vi "AssembleBLMultiplotScript-UandTI.vi"(0 "name or relative path":string, 1 "Final Title":string, 2 "Spectra?":bool, 3 "NormaliseHeight?":bool, 4 "Zref":dbl, 5 "Fit Zmax":dbl, 6 "Fit Zmin":dbl, 7 "HeightJitter%":dbl, 8 "Scale":dbl, 9 "BL Targets":T2[](array[typedef]) {"n" min=0.02 max=0.5 step=0.01 format="%.2f"}, 10 "U,L(U)":refnum<vi>, 11 "UtargetsInfo":T1(array[cluster]), 12 "TI,Sigma":refnum<vi>, 13 "TItargetsInfo":T1(array[cluster]), 15 "No d0":cluster{"n":dbl, "d0":dbl, "d0 2":dbl}, 17 "with d0":cluster{"n":dbl, "d0":dbl, "d0 2":dbl}) -> (20 "gnuplotOut":string)   [LabVIEW 2014]
uses:
  EnFloSFCPPHybrid/Anemometry/Anemometry Sub Vis/Data_plotting_vis/gnuplotScriptComponents/BLPlottersubVIs/BLTarget.ctl
  EnFloSFCPPHybrid/Anemometry/Anemometry Sub Vis/Data_plotting_vis/gnuplotScriptComponents/at.ctl
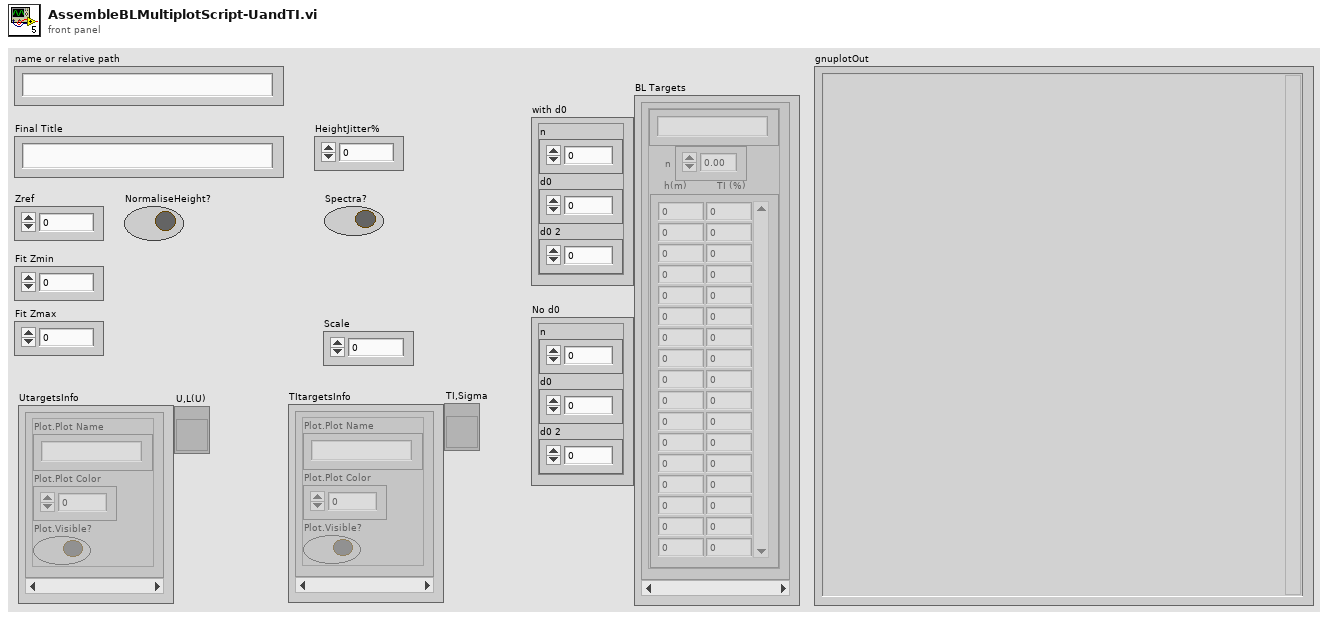
[diagram p1: front panel]
types:
  T1 = cluster{"Plot.Plot Name":string, "Plot.Plot Color":u32, "Plot.Visible?":bool}[]
  T2 = typedef "BLTarget.ctl" = cluster{"Code":string, "TI Profile (FS)":dbl[][], "n":dbl}
  T3 = typedef "at.ctl" = cluster{"XcoordSys":string, "YcoordSys":string, "Xvalue":dbl, "Yvalue":dbl}
  T4 = typedef "minAndMax.ctl" = cluster{"Min":T5, "Max":T5}
  T5 = typedef "AutoManualNumber.ctl" = cluster{"Auto":bool, "Value":dbl}
  T6 = cluster{"No d0":cluster{"n":dbl, "d0":dbl, "d0 2":dbl}, "with d0":cluster{"n":dbl, "d0":dbl, "d0 2":dbl}}
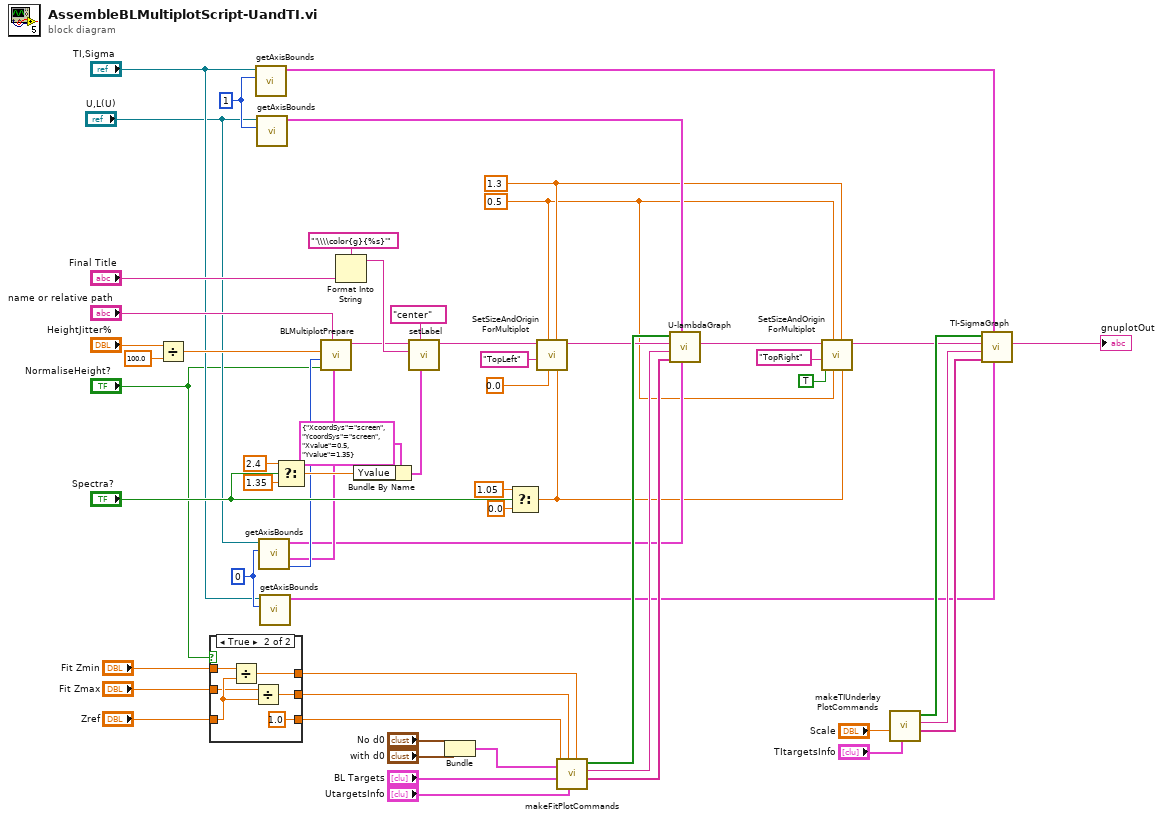
[diagram p0: block diagram]
diagram:
  w16 = 0.5 ("IndividualWidth")
  w17 = 1.3 ("IndividualHeight")
  w11 = 1 ("Active X Scale")
  w10 = 0 ("Active X Scale")
  n1 = Divide(x="HeightJitter%", y=100.0) -> (x/y=w28:dbl)
  n2 = case shown="True" "NormaliseHeight?" {
    tunnel: "Fit Zmin" -> [w62 w68]
    tunnel: "Zref" -> [w60 w67]
    tunnel: "Fit Zmax" -> [w61 w66]
    tunnel: [w62 w65] -> w3
    tunnel: [w61 w64] -> w2
    tunnel: [w60 1.0 ("Zref")] -> w1
    frame False {
    }
    frame True {
      n3 = Divide(x=w68, y=w67) -> (x/y=w65:dbl)
      n4 = Divide(x=w66, y=w67) -> (x/y=w64:dbl)
    }
  }
  n5 = call "getAxisBounds.vi"("Active X Scale"=w11, "XYGraph in"="TI,Sigma") -> ("Xbounds"=w23:T4)  [unwired: 6 in, 3 out]
  n6 = call "getAxisBounds.vi"("Active X Scale"=w11, "XYGraph in"="U,L(U)") -> ("Xbounds"=w25:T4)  [unwired: 6 in, 3 out]
  n7 = call "getAxisBounds.vi"("Active X Scale"=w10, "XYGraph in"="U,L(U)") -> ("YMapping"=w31:enum8{"Lin", "Log"}, "Ybounds"=w30:T4, "Xbounds"=w26:T4)  [unwired: 6 in, 1 out]
  n8 = call "getAxisBounds.vi"("Active X Scale"=w10, "XYGraph in"="TI,Sigma") -> ("Xbounds"=w27:T4)  [unwired: 6 in, 3 out]
  n9 = Select(t=2.4 ("Yvalue"), s="Spectra?", f=1.35 ("Yvalue")) -> (s? t:f=w56:dbl)
  n10 = call "BLMultiplotPrepare.vi"("HeightAxisBounds"=w30, "ProfileFilename"="name or relative path", "NormaliseHeight?"="NormaliseHeight?", "YaxisMapping"=w31, "jitterFraction"=w28) -> ("gnuplotOut"=w33:string)  [unwired: 6 in]
  n11 = Format Into String(format string="'\\\\color{g}{%s}'" ("string"), "Final Title") -> (resulting string=w38:string)  [unwired: 2 in, 1 out]
  n12 = Bundle By Name(cluster=T3 {"XcoordSys"="screen", "YcoordSys"="screen", "Xvalue"=0.5, "Yvalue"=1.35} ("\"At\" location"), "Yvalue"=w56) -> (w52:T3)
  n13 = call "setLabel.vi"("\"At\" location"=w52, "Justify"="center" ("Horizontal"), "singleLabel"=w38, "String in"=w33) -> ("String out"=w34:string)  [unwired: 6 in, 1 out]
  n14 = Bundle("No d0"="No d0", "with d0"="with d0") -> (w44:T6)  [unwired: 1 in]
  n15 = Select(t=1.05, s="Spectra?", f=0.0) -> (s? t:f=w24:dbl)
  n16 = call "SetSizeAndOriginForMultiplot.vi"("VerticalPosition"=w24, "Height"=w17, "LateralPosition"=0.0, "Width"=w16, "PlotLocationDescription"="TopLeft", "gnuplotIn"=w34) -> ("gnuplotOut"=w22:string)  [unwired: 5 in]
  n17 = call "makeFitPlotCommands.vi"("Fit Zmin"=w3, "plotInfoArray"="UtargetsInfo", "Fit Zmax"=w2, "BL Targets"="BL Targets", "Coefficients"=w44, "Zref"=w1) -> ("UnderlayPlotSeries"=w40:string[], "Pre-plot Injection"=w39:string, "BasicsVisible"=w58:bool[])  [unwired: 3 in]
  n18 = call "U-lambdaGraph.vi"("U/Uref bounds"=w26, "lambda bounds"=w25, "UnderlayPlotSeries"=w40, "Pre-plot Injection"=w39, "gnuplotIn"=w22, "BasicsVisible"=w58) -> ("gnuplotOut"=w41:string)  [unwired: 5 in]
  n19 = call "SetSizeAndOriginForMultiplot.vi"("VerticalPosition"=w24, "Height"=w17, "LateralPosition"=w16, "Width"=w16, "ClearLabels?"=TRUE, "PlotLocationDescription"="TopRight", "gnuplotIn"=w41) -> ("gnuplotOut"=w18:string)  [unwired: 4 in]
  n20 = call "makeTIUnderlayPlotCommands.vi"("plotInfoArray"="TItargetsInfo", "Scale"="Scale") -> ("UnderlayPlotSeries"=w48:string[], "Pre-plot Injection"=w50:string, "Basics Visible"=w59:bool[])  [unwired: 7 in]
  n21 = call "TI-SigmaGraph.vi"("TI bounds"=w27, "sigma/U bounds"=w23, "UnderlayPlotSeries"=w48, "Pre-plot Injection"=w50, "gnuplotIn"=w18, "Basics Visible"=w59) -> ("gnuplotOut"=→"gnuplotOut":string)  [unwired: 5 in]
